vi "Set Shifter (Bool).vi"(8 "error in (no error)":errorcluster, 10 "Low":bool, 11 "High":bool) -> (0 "error out":errorcluster)   [LabVIEW 2011]
uses:
  Shared/Shifter State.ctl
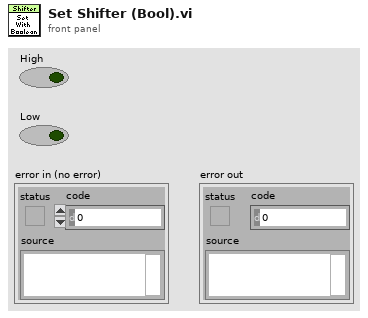
[diagram p1: front panel]
types:
  T1 = typedef "Shifter State.ctl" = enum16{"Unknown", "Low", "High"}
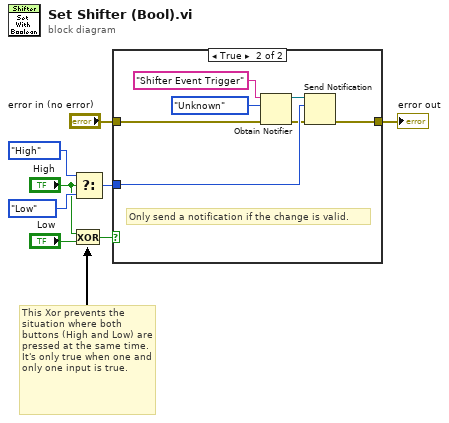
[diagram p0: block diagram]
diagram:
  # "This Xor prevents the situation where both buttons (High and Low) are pressed at the same time.  It's only true when one and only one input is true."
  n1 = Exclusive Or(1:"Low", 2:"High") -> (0:w3:bool)
  n2 = Select(t=Shifter_State."High", s="High", f=Shifter_State."Low") -> (s? t:f=w4:T1)
  n3 = case shown="True" w3 {
    tunnel: w4 -> [_ w13]
    tunnel: "error in (no error)" -> [w9 w11]
    tunnel: [w9 w10] -> w6
    frame False {
    }
    frame True {
      # "Only send a notification if the change is valid."
      n4 = Obtain Notifier(name (unnamed)="Shifter Event Trigger", notification data type=Shifter_State."Unknown", error in (no error)=w11) -> (notifier out=w14:refnum<notifier>, error out=w12:errorcluster)  [unwired: 1 in, 1 out]
      n5 = Send Notification(notification=w13, notifier=w14, error in (no error)=w12) -> (error out=w10:errorcluster)  [unwired: 1 out]
    }
  }
  "error out" <- w6
